vi "Radar_4channel_DAQ.vi"() -> ()   [LabVIEW 2015]
doc: "Personal Daq 54 example.\nTriggering is immediate and readings are returned 1 scan at a time as available.\nBe sure to use the Acquisition Stop control for proper shutdown."
uses:
  <vilib>/Utility/error.llb/DialogType.ctl
  <vilib>/DAQmx/read.llb/DAQmx Read (Analog 1D DBL NChan 1Samp).vi
  <vilib>/Analysis/2dsp.llb/Complex FFT.vi
  <vilib>/DAQmx/create/channels.llb/DAQmx Create Channel (AI-Voltage-Basic).vi
  <vilib>/DAQmx/configure/timing.llb/DAQmx Timing (Sample Clock).vi
  <vilib>/DAQmx/miscellaneous.llb/DAQmx Fill In Error Info.vi
  <vilib>/measure/madcrms.llb/Basic Averaged DC-RMS for 1 Chan.vi
  <vilib>/measure/NI_MAPro.lvlib
  <vilib>/Analysis/NI_AALPro.lvlib
panel:
  in  "CH2 Q channel":i32=3
  in  "CH2 I channel":i32=2
  in  "CH1 Q channel":i32=1
  in  "CH1 I channel":i32
  in  "FFT length":i32=2048
  in  "buffer size":i32=256
  in  "samples per channel":i32=1
  in  "rate":dbl=20.0 format="%0.2f"
  in  "input terminal":i32(ring)=10083 items=["Default"=-1, "RSE"=10083, "NRSE"=10078, "Differential"=10106, "Pseudodifferential"=12529]
  in  "minimum value":dbl format="%0.2f"
  in  "maximum value":dbl=5.0 format="%0.2f"
  out "Spectrum 2":waveform(dbl)(graph)
  out "I/Q Signal 2":dynamicdata(graph)
  out "I/Q Signal 1":dynamicdata(graph)
  in  "Save Data":bool
  in  "stop":bool
  out "Spectrum 1":waveform(dbl)(graph)
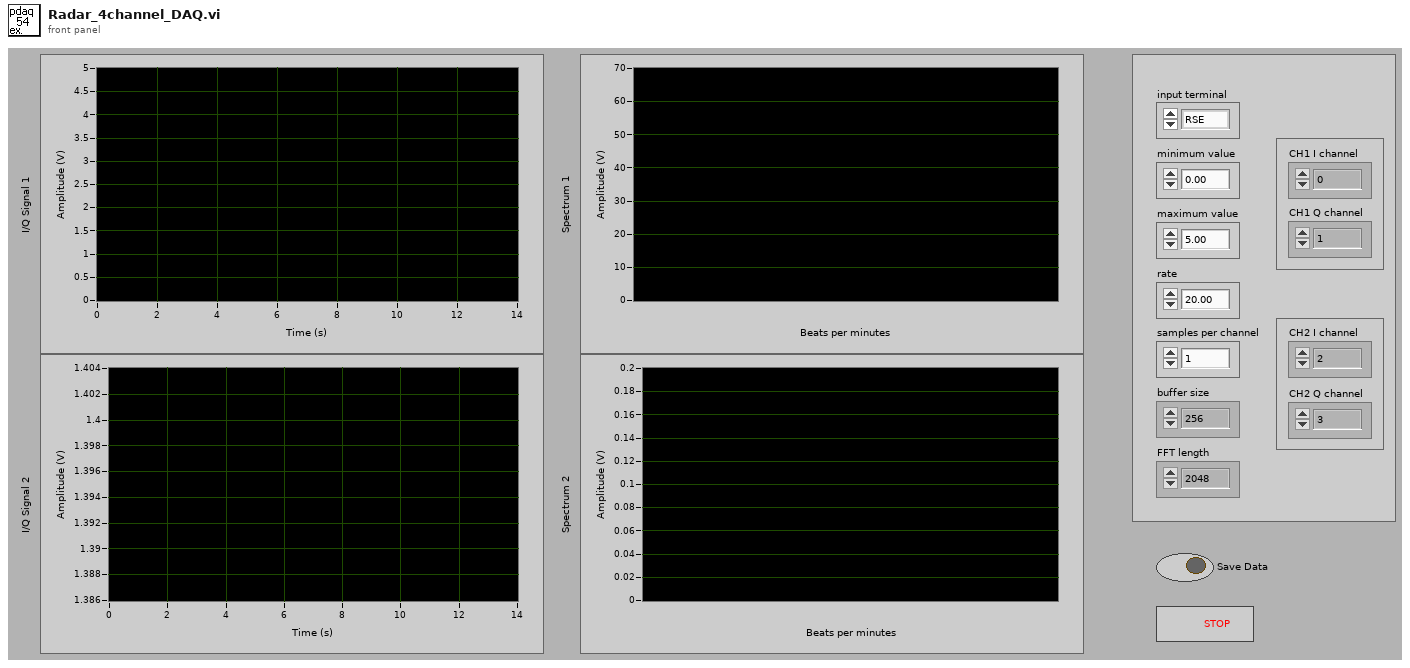
[diagram p1: front panel]
types:
  T1 = typedef "DialogType.ctl" = u16
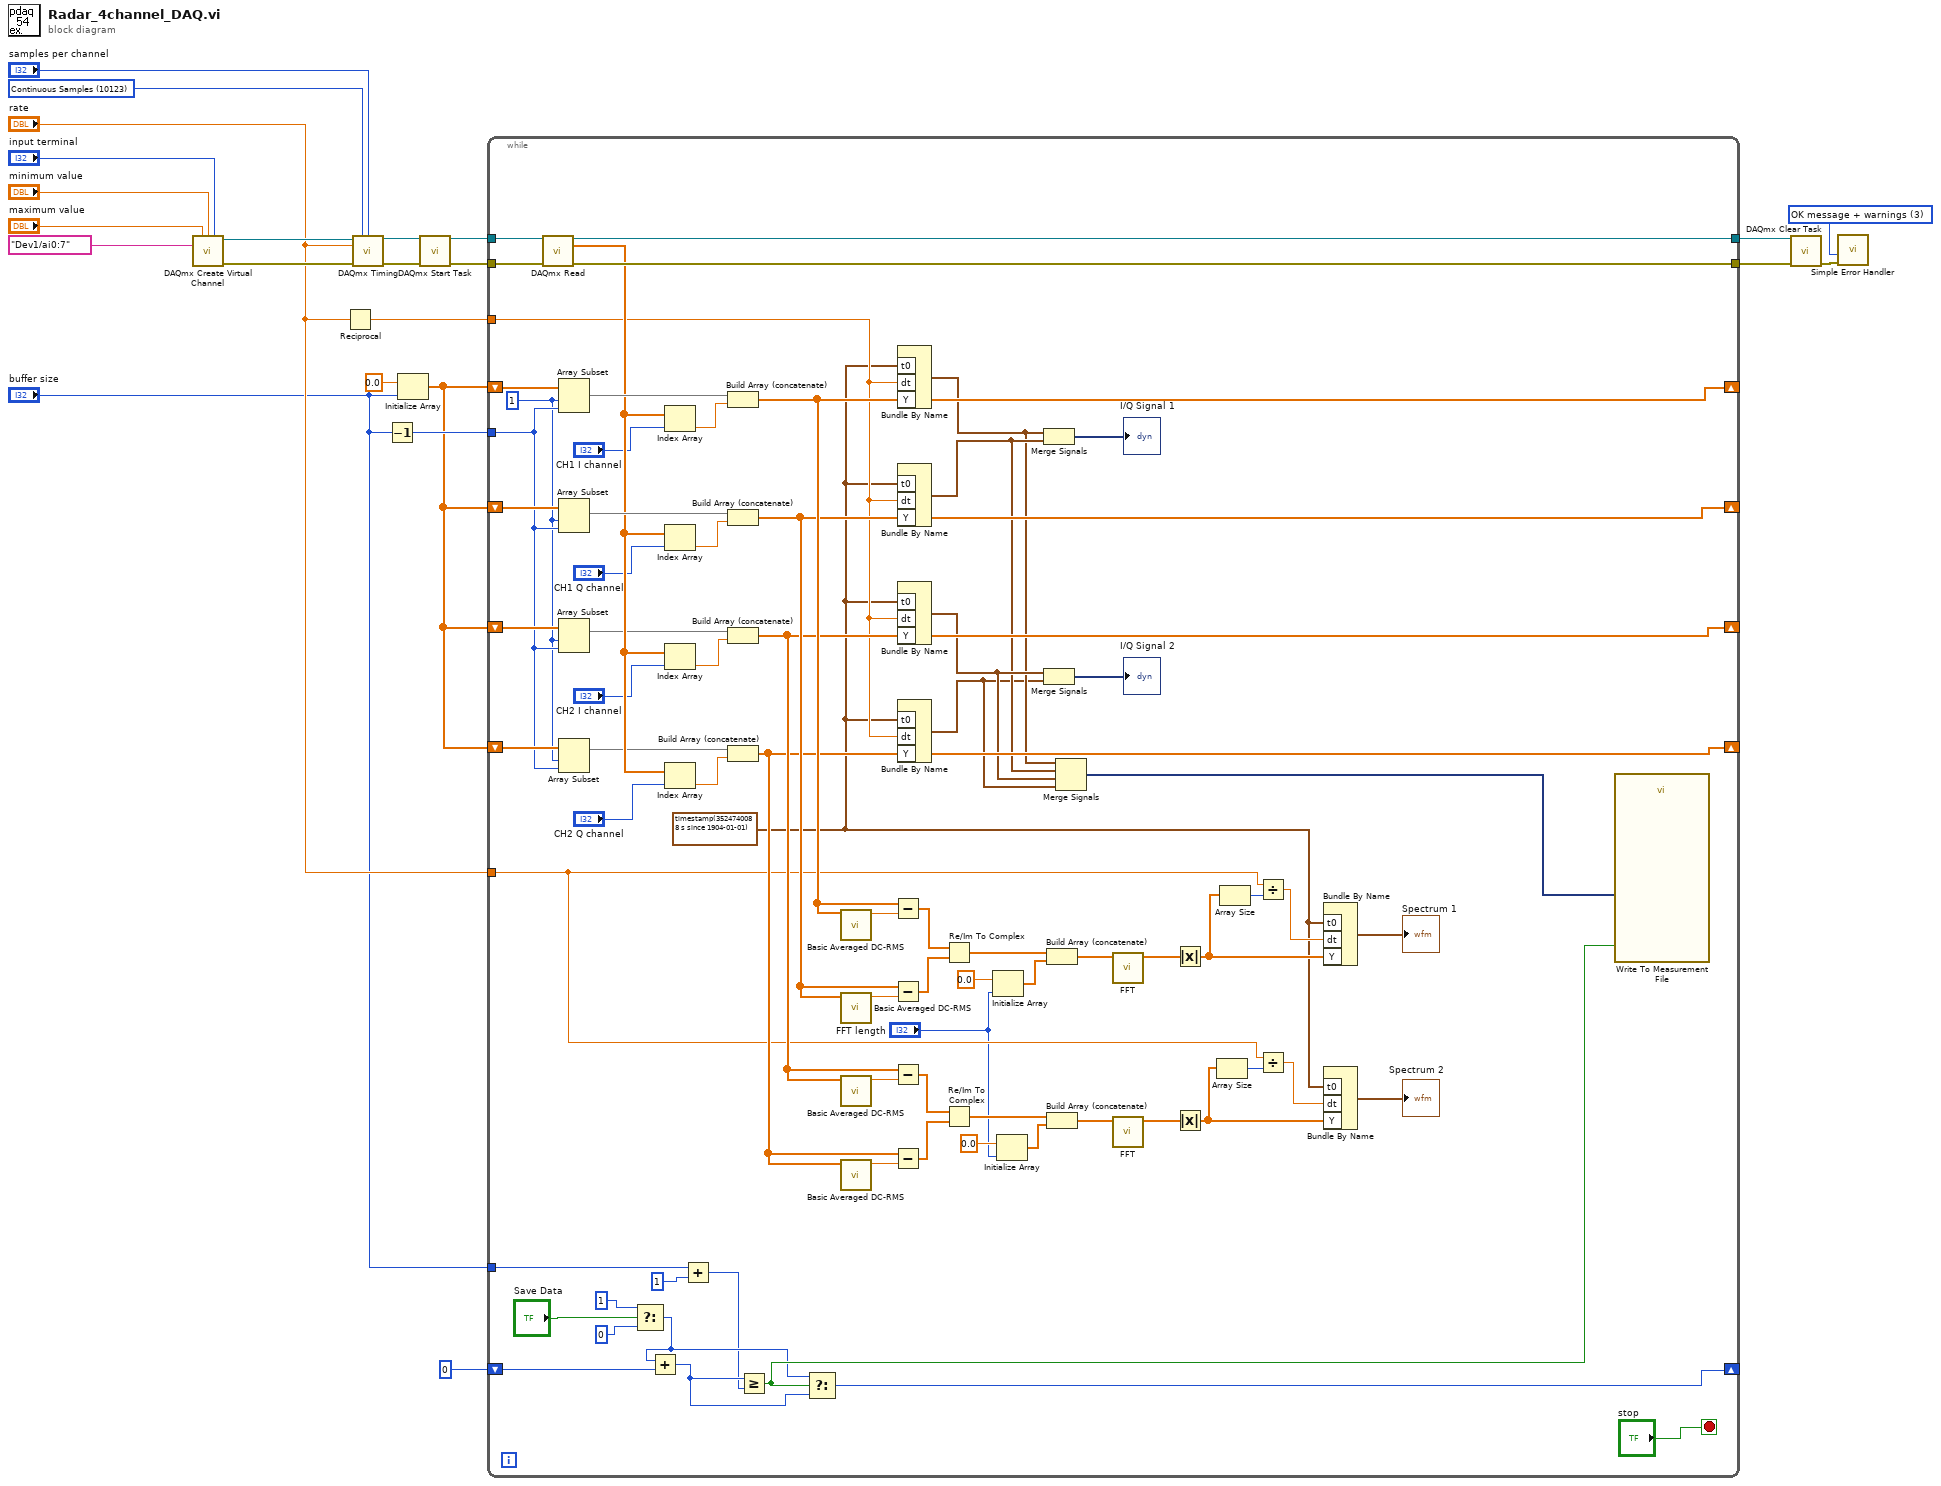
[diagram p0: block diagram]
diagram:
  w14 = T1 3 items=["no dialog", "OK message", "continue or stop message", "OK message + warnings", "continue/stop + warnings"] ("type of dialog (OK msg:1)")
  w7 = 10123 items=["Finite Samples"=10178, "Continuous Samples"=10123] ("sample mode")
  n1 = call-poly <vilib>:"DAQmx Create Virtual Channel.vi"("maximum value"="maximum value", "minimum value"="minimum value", "input terminal configuration"="input terminal", "physical channels"=tag "Dev1/ai0:7") -> ("task out"=w20:refnum<k21>, "error out"=w21:errorcluster)  [unwired: 5 in, 5 out]
  n2 = Reciprocal(x="rate") -> (1/x=w8:dbl)
  n3 = call-poly <vilib>:"DAQmx Timing.vi"("task/channels in"=w20, "sample mode"=w7, "samples per channel"="samples per channel", "rate"="rate", "error in"=w21) -> ("task out"=w19:refnum<k21>, "error out"=w18:errorcluster)  [unwired: 2 in, 7 out]
  n4 = Decrement(x="buffer size") -> (x-1=w22:i32)
  n5 = Initialize Array(0.0 ("element"), "buffer size") -> (w9:dbl[])
  n6 = call <vilib>:"DAQmx Start Task.vi"("task/channels in"=w19, "error in"=w18) -> ("task out"=w16:refnum<k21>, "error out"=w15:errorcluster)  [unwired: 12 out]
  n7 = while {
    shift-right: [w88] -> _
    shift-left: w9 -> [w99]
    tunnel: w22 -> [w66]
    shift-right: [w87] -> _
    shift-left: w9 -> [w97]
    tunnel: w16 -> [w86]
    tunnel: w15 -> [w85]
    tunnel: w8 -> [w34]
    tunnel: [w84] -> w13
    tunnel: [w83] -> w12
    tunnel: "buffer size" -> [w32]
    shift-right: [w75] -> _
    shift-left: 0 -> [w77]
    shift-right: [w59] -> _
    shift-left: w9 -> [w68]
    shift-right: [w58] -> _
    shift-left: w9 -> [w67]
    tunnel: "rate" -> [w30]
    stop <- "stop" stop-if-true
    w33 = timestamp(3524740088.296 s since 1904-01-01) ("t0")
    w29 = 1 ("index")
    n8 = call-poly <vilib>:"DAQmx Read.vi"("task/channels in"=w86, "error in"=w85) -> ("task out"=w84:refnum<k21>, "data"=w65:dbl[], "error out"=w83:errorcluster)  [unwired: 11 out]
    n9 = Array Subset(array=w99, index=w29, length=w66) -> (w98:dbl[])
    n10 = Array Subset(array=w97, index=w29, length=w66) -> (w96:dbl[])
    n11 = Array Subset(array=w68, index=w29, length=w66) -> (w35:dbl[])
    n12 = Array Subset(array=w67, index=w29, length=w66) -> (w64:dbl[])
    n13 = Select(t=1, s="Save Data", f=0) -> (s? t:f=w71:i32)
    n14 = Add(x=w71, y=w77) -> (x+y=w76:i32)
    n15 = Index Array(array=w65, index="CH1 I channel") -> (element=w39:dbl)
    n16 = Index Array(array=w65, index="CH1 Q channel") -> (element=w38:dbl)
    n17 = Index Array(array=w65, index="CH2 I channel") -> (element=w37:dbl)
    n18 = Index Array(array=w65, index="CH2 Q channel") -> (element=w36:dbl)
    n19 = Add(x=w32, y=1 ("index")) -> (x+y=w62:i32)
    n20 = Build Array (concatenate)(w98, w39) -> (w88:dbl[])
    n21 = Build Array (concatenate)(w96, w38) -> (w87:dbl[])
    n22 = Build Array (concatenate)(w35, w37) -> (w59:dbl[])
    n23 = Build Array (concatenate)(w64, w36) -> (w58:dbl[])
    n24 = Greater Or Equal?(x=w76, y=w62) -> (x >= y?=w74:bool)
    n25 = Select(t=w71, s=w74, f=w76) -> (s? t:f=w75:i32)
    n26 = call-poly <vilib>:"Basic Averaged DC-RMS.vi"("signal in"=w88) -> ("DC value"=w92:dbl)  [unwired: 4 in, 6 out]
    n27 = call-poly <vilib>:"Basic Averaged DC-RMS.vi"("signal in"=w87) -> ("DC value"=w93:dbl)  [unwired: 4 in, 6 out]
    n28 = call-poly <vilib>:"Basic Averaged DC-RMS.vi"("signal in"=w59) -> ("DC value"=w60:dbl)  [unwired: 4 in, 6 out]
    n29 = call-poly <vilib>:"Basic Averaged DC-RMS.vi"("signal in"=w58) -> ("DC value"=w61:dbl)  [unwired: 4 in, 6 out]
    n30 = Subtract(x=w88, y=w92) -> (x-y=w81:dbl[])
    n31 = Subtract(x=w87, y=w93) -> (x-y=w80:dbl[])
    n32 = Subtract(x=w59, y=w60) -> (x-y=w56:dbl[])
    n33 = Subtract(x=w58, y=w61) -> (x-y=w57:dbl[])
    n34 = Bundle By Name("t0"=w33, "dt"=w34, "Y"=w88) -> (w50:waveform(dbl))  [unwired: 1 out]
    n35 = Bundle By Name("t0"=w33, "dt"=w34, "Y"=w87) -> (w51:waveform(dbl))  [unwired: 1 out]
    n36 = Bundle By Name("t0"=w33, "dt"=w34, "Y"=w59) -> (w52:waveform(dbl))  [unwired: 1 out]
    n37 = Bundle By Name("t0"=w33, "dt"=w34, "Y"=w58) -> (w31:waveform(dbl))  [unwired: 1 out]
    n38 = Re/Im To Complex(1:w80, 2:w81) -> (0:w94:cdb[])
    n39 = Re/Im To Complex(1:w57, 2:w56) -> (0:w40:cdb[])
    n40 = Initialize Array(0.0 ("element"), "FFT length") -> (w55:dbl[])
    n41 = Initialize Array(0.0 ("element"), "FFT length") -> (w48:dbl[])
    n42 = Merge Signals(w50, w51) -> (→"I/Q Signal 1":dynamicdata)
    n43 = Merge Signals(w52, w31) -> (→"I/Q Signal 2":dynamicdata)
    n44 = Build Array (concatenate)(w94, w55) -> (w89:cdb[])
    n45 = Build Array (concatenate)(w40, w48) -> (w44:cdb[])
    n46 = Merge Signals(w50, w51, w52, w31) -> (w49:dynamicdata)
    n47 = call-poly <vilib>:"FFT.vi"("X"=w89) -> ("FFT {X}"=w91:cdb[])  [unwired: 2 in, 8 out]
    n48 = call-poly <vilib>:"FFT.vi"("X"=w44) -> ("FFT {X}"=w42:cdb[])  [unwired: 2 in, 8 out]
    n49 = Absolute Value(x=w91) -> (abs(x)=w69:dbl[])
    n50 = Absolute Value(x=w42) -> (abs(x)=w47:dbl[])
    n51 = Array Size(array=w47) -> (size(s)=w43:i32)
    n52 = Array Size(array=w69) -> (size(s)=w90:i32)
    n53 = Divide(x=w30, y=w90) -> (x/y=w78:dbl)
    n54 = Divide(x=w30, y=w43) -> (x/y=w46:dbl)
    n55 = Bundle By Name("t0"=w33, "dt"=w78, "Y"=w69) -> (→"Spectrum 1":waveform(dbl))  [unwired: 1 out]
    n56 = Bundle By Name("t0"=w33, "dt"=w46, "Y"=w47) -> (→"Spectrum 2":waveform(dbl))  [unwired: 1 out]
    n57 = call "Write To Measurement File"("Signals"=w49, "Enable"=w74) -> ()  [unwired: 15 in, 3 out]
  }
  n58 = call <vilib>:"DAQmx Clear Task.vi"("task in"=w13, "error in"=w12) -> ("error out"=w11:errorcluster)  [unwired: 13 out]
  n59 = call <vilib>:"Simple Error Handler.vi"("type of dialog (OK msg:1)"=w14, "error in (no error)"=w11) -> ()  [unwired: 8 out]
